vi "BCtr6.vi"() -> ()   [LabVIEW 2016]
uses:
  <vilib>/Platform/TimedLoop/XDataNode/timing_clust.ctl
  <vilib>/Platform/TimedLoop/XDataNode/nitl_modes.ctl
  <vilib>/Platform/TimedLoop/XDataNode/wakeup.ctl
  <vilib>/platform/TimedLoop/XDataNode/XDataNode.xnode
  <vilib>/Platform/TimedLoop/XDataNode/XDNodeRunTimeDep.lvlib
panel:
  in  "stop":bool
  out "Waveform Chart":u16(graph)
  out "LoopCt":dbl
  out "Ack":bool
  out "error out":errorcluster
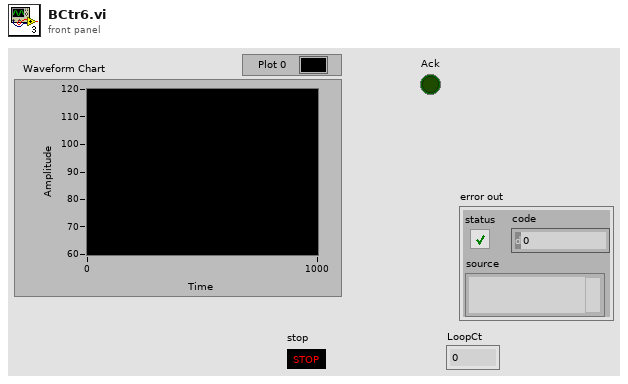
[diagram p1: front panel]
types:
  T1 = cluster{"Nbins":u16, "BaseAddrOut":u16, "PortOut":string, "ConfigOK":bool, "MreadFmt":string}
  T2 = typedef "XDNodeRunTimeDep.lvlib/timing_clust.ctl" = cluster{"Expected End [f-1]":u64, "Actual End [f-1]":u64, "Finished Late? [f-1]":bool, "Expected End [i-1]":u64, "Actual End [i-1]":u64, "Finished Late? [i-1]":bool, "Expected Start [i]":u64, "Actual Start [i]":u64, "Expected Start [f]":u64, "Actual Start [f]":u64, "Source Name":string, "Structure Name":string, "Period":i64, "Deadline":i64, "Offset":i64, "Start":i64, "Priority":i32, "Timeout":i32, "Mode":T3, "Wakeup Reason":T4, "Error":errorcluster, "Source Type":string, "Secondary Source Type":string, "Global End Time":u64, "Global Start Time":u64, "Frame Duration":u64, "Iteration Duration":u64, "Assigned CPU":i32, "I/O Scan Engine Mode":u32}
  T3 = typedef "XDNodeRunTimeDep.lvlib/nitl_modes.ctl" = enum32{"No Change", "Process missed periods, maintain original phase", "Discard missed periods, maintain original phase", "Process missed periods, ignore original phase", "Discard missed periods, ignore original phase"}
  T4 = typedef "XDNodeRunTimeDep.lvlib/wakeup.ctl" = enum32{"Normal", "Aborted", "Asynchronous wakeup", "Timing source error", "Timed loop error", "Timeout"}
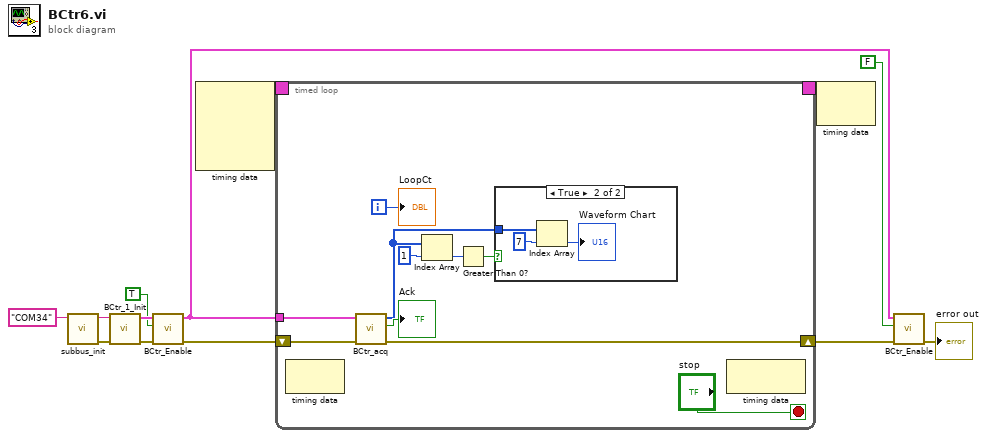
[diagram p0: block diagram]
diagram:
  n1 = call "subbus_init.vi"("Port"="COM34") -> ("error out"=w9:errorcluster, "PortOut"=w10:string)  [unwired: 9 in]
  n2 = call "BCtr_1_Init.vi"("error in (no error)"=w9, "SBPort"=w10) -> ("error out"=w7:errorcluster, "CtrCfg"=w8:T1)  [unwired: 8 in]
  n3 = call "BCtr_Enable.vi"("error in (no error)"=w7, "Enable"=TRUE, "CtrCfg"=w8) -> ("error out"=w6:errorcluster, "CtrCfgOut"=w2:T1)  [unwired: 5 in, 1 out]
  n4 = node-c288() -> (w12:T2)  [unwired: 4 in]
  n5 = timed-loop {
    timing: w12 -> [_]
    timing-out: [_] -> w11
    shift-right: [w22] -> w4
    shift-left: w6 -> [w23]
    tunnel: w2 -> [w15]
    i -> [w20]
    stop <- "stop" stop-if-true
    n6 = node-c288() -> ()  [unwired: 1 in, 1 out]
    n7 = call "BCtr_acq.vi"("error in (no error)"=w23, "CtrCfg"=w15) -> ("error out"=w22:errorcluster, "Ack"=→"Ack":bool, "Values"=w19:u16[])  [unwired: 7 in]
    n8 = Index Array(array=w19, index=1) -> (element=w17:u16)
    n9 = Greater Than 0?(x=w17) -> (x > 0?=w16:bool)
    n10 = case shown="True" w16 {
      tunnel: w19 -> [_ w26]
      frame False {
      }
      frame True {
        n11 = Index Array(array=w26, index=7) -> (element=→"Waveform Chart":u16)
      }
    }
    n12 = node-c288() -> ()  [unwired: 1 in, 1 out]
    "LoopCt" <- w20
  }
  n13 = node-c288(w11) -> ()  [unwired: 1 out]
  n14 = call "BCtr_Enable.vi"("error in (no error)"=w4, "Enable"=FALSE, "CtrCfg"=w2) -> ("error out"=→"error out":errorcluster)  [unwired: 5 in, 2 out]
